vi "Copilots Controller Init.vi"(8 "error in":errorcluster) -> (0 "error out":errorcluster)   [LabVIEW 2015]
uses:
  <vilib>/Rock Robotics/WPI/Joystick/WPI_JoystickDeviceEnum.ctl
  Support/Global Objects.vi
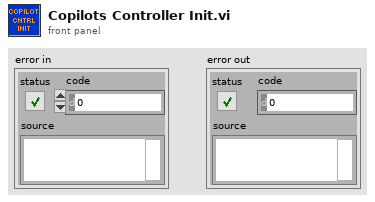
[diagram p1: front panel]
types:
  T1 = typedef "Joystick Info.ctl" = cluster{"JoystickDevRef":T2}
  T2 = typedef "WPI_JoystickDevRef.ctl" = cluster{"Device":T3}
  T3 = typedef "WPI_JoystickDeviceEnum.ctl" = enum16{"USB 0", "USB 1", "USB 2", "USB 3", "USB 4", "USB 5"}
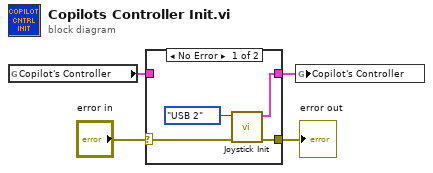
[diagram p0: block diagram]
diagram:
  n1 = global read "Global Objects.vi" "Copilot's Controller"() -> (w2:T1)
  n2 = case shown="No Error" "error in" {
    selector: "error in" -> [w6 w10]
    tunnel: [w5 w10] -> w3
    tunnel: [w7 w9] -> w1
    tunnel: w2 -> [_ w9]
    frame No Error {
      n3 = call "Joystick Init.vi"("error in"=w6, "JoystickDevice"=WPI_JoystickDeviceEnum."USB 2") -> ("error out"=w5:errorcluster, "Joystick Out"=w7:T1)  [unwired: 8 in]
    }
    frame Error {
    }
  }
  "error out" <- w3
  n4 = global write "Global Objects.vi" "Copilot's Controller"(w1) -> ()
